vi "Write.vi"(8 "error in":errorcluster, 10 "Data In":string, 11 "Serial Session in":refnum<class "Serial Session.lvclass">) -> (0 "error out":errorcluster, 3 "Serial Session out":refnum<class "Serial Session.lvclass">)   [LabVIEW 2015, in "Serial Session.lvclass"]
doc: "Asynchronous write to port."
uses:
  Serial Session.lvclass
  Serial Session.lvclass/Serial Session.ctl
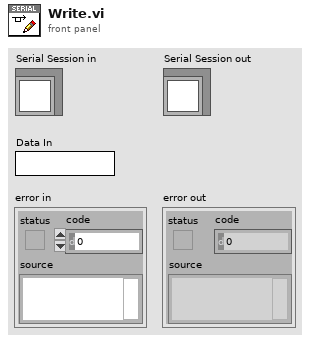
[diagram p1: front panel]
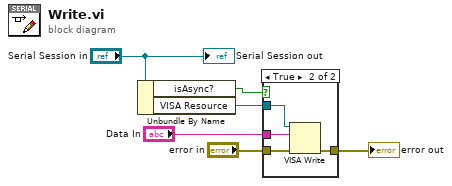
[diagram p0: block diagram]
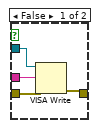
[diagram p2: hidden frame]
diagram:
  n1 = Unbundle By Name("Serial Session in") -> ("isAsync?"=w1:bool, "VISA Resource"=w5:refnum<visa-resource-name>)
  n2 = case shown="True" w1 {
    tunnel: w5 -> [w10 w14]
    tunnel: "Data In" -> [w9 w13]
    tunnel: "error in" -> [w8 w12]
    tunnel: [w7 w11] -> w2
    frame False {
      n3 = VISA Write(VISA resource name=w10, write buffer=w9, error in (no error)=w8) -> (error out=w7:errorcluster)  [unwired: 2 out]
    }
    frame True {
      n4 = VISA Write(VISA resource name=w14, write buffer=w13, error in (no error)=w12) -> (error out=w11:errorcluster)  [unwired: 2 out]
    }
  }
  "error out" <- w2
  "Serial Session out" <- "Serial Session in"
